vi "Organizing Tool.vi"() -> ()   [LabVIEW 2024]
uses:
  <userlib>/_OpenG.lib/file/file.llb/openg_file.lvlib
panel:
  in  "dest folders":i32(listbox)
  in  "root path":path
  in  "source folders":i32(listbox)
  in  "Delete Source Only":bool
  in  "Copy from Source":bool
  in  "Delete Source Dir?":bool=TRUE
  in  "Move and Delete Source":bool
  in  "dest files":i32(listbox)
  in  "source files":i32(listbox)
  in  "Quit":bool
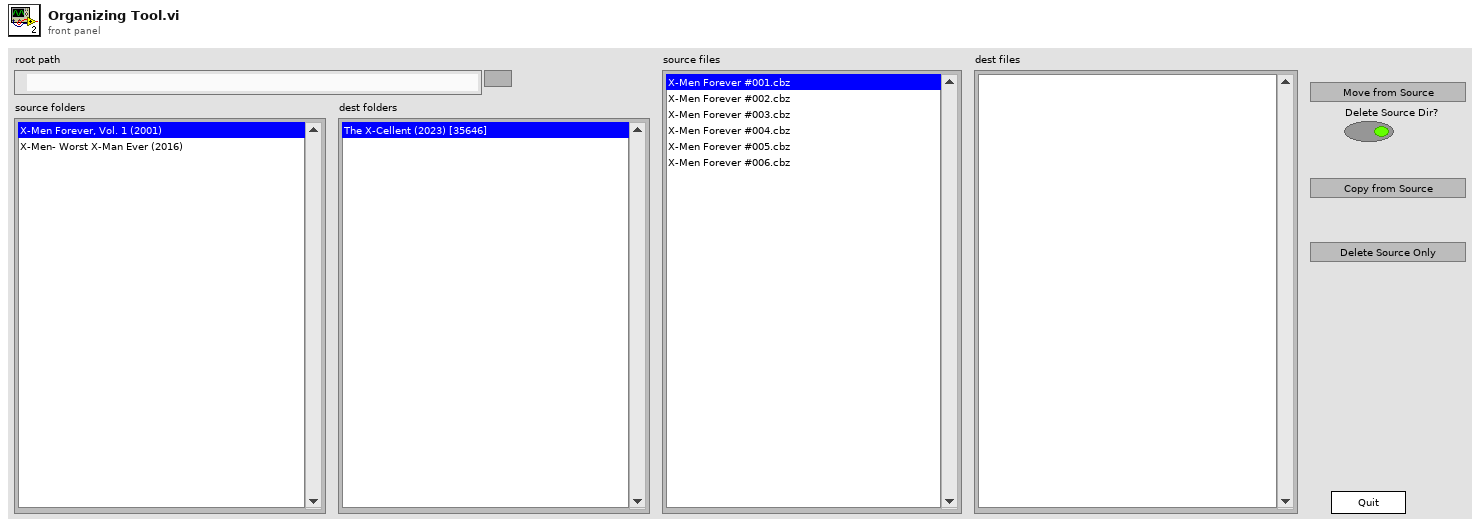
[diagram p1: front panel]
types:
  T1 = enum32{"Invalid", "Standard", "Closed", "Hidden", "Minimized", "Maximized"}
  T2 = enum32{"invalid app kind", "Development System", "Run Time System", "Student Edition", "Embedded LabVIEW", "Evaluation", "Custom"}
  T3 = cluster{"Core":cluster{"Current VI Reference":refnum<vi>, "Close Panel on Exit?":bool}, "source path":path, "dest path":path, "last source value":i32, "last dest value":i32}
  T4 = cluster{"Current VI Reference":refnum<vi>, "Close Panel on Exit?":bool}
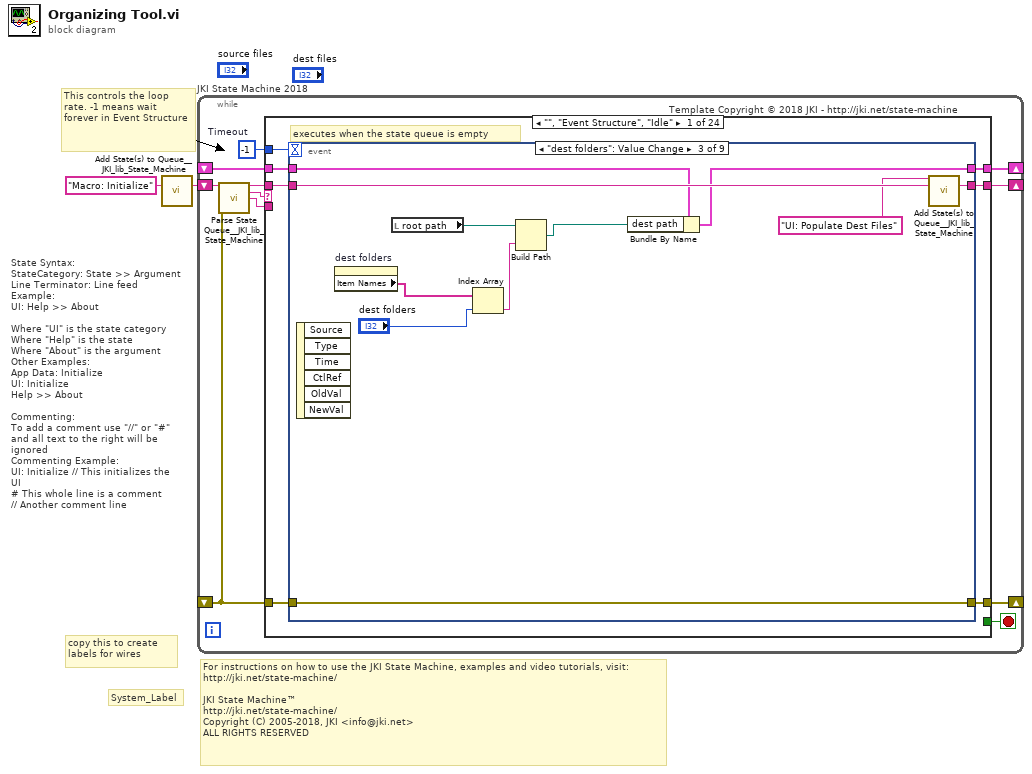
[diagram p0: block diagram]
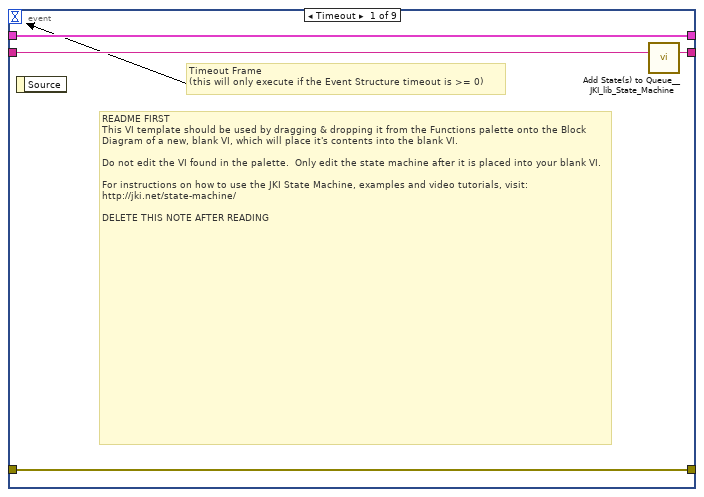
[diagram p2: hidden frame]
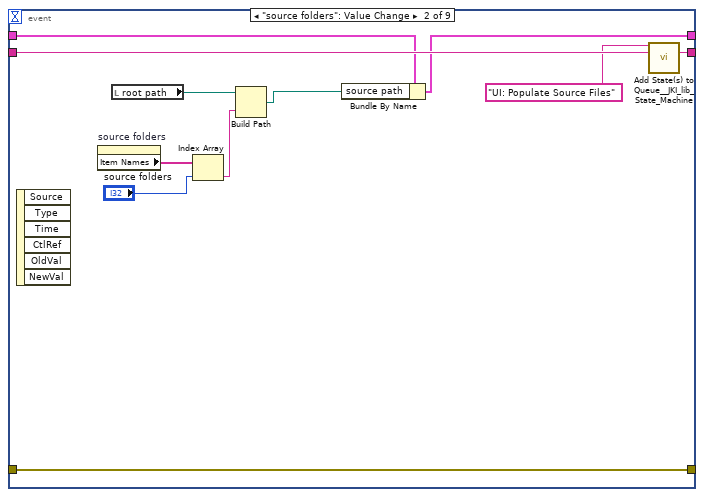
[diagram p3: hidden frame]
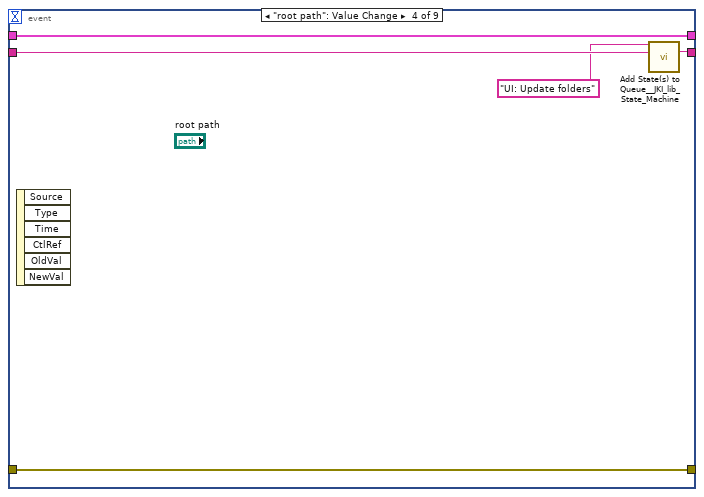
[diagram p4: hidden frame]
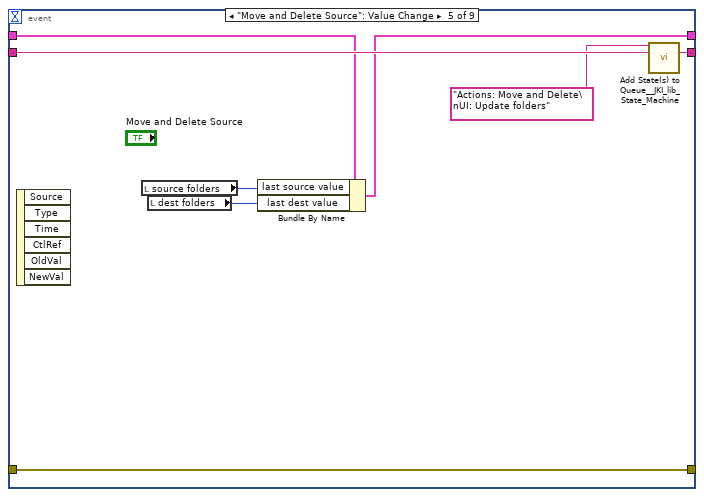
[diagram p5: hidden frame]
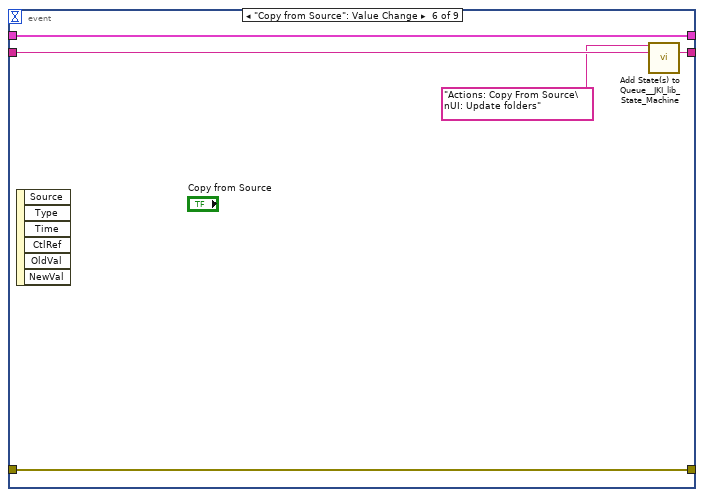
[diagram p6: hidden frame]
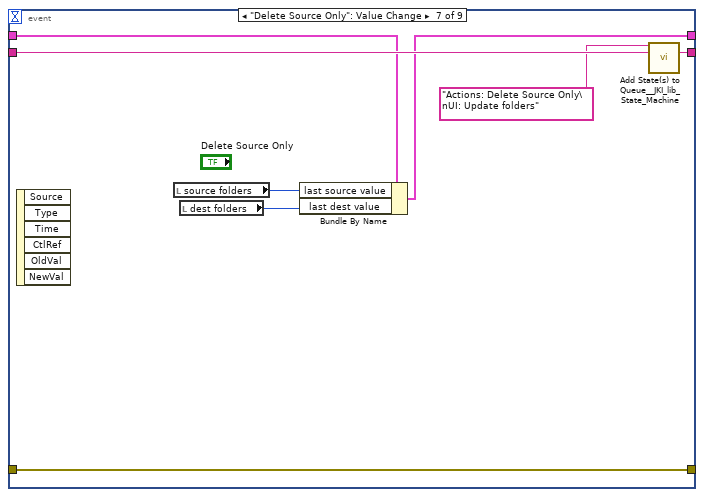
[diagram p7: hidden frame]
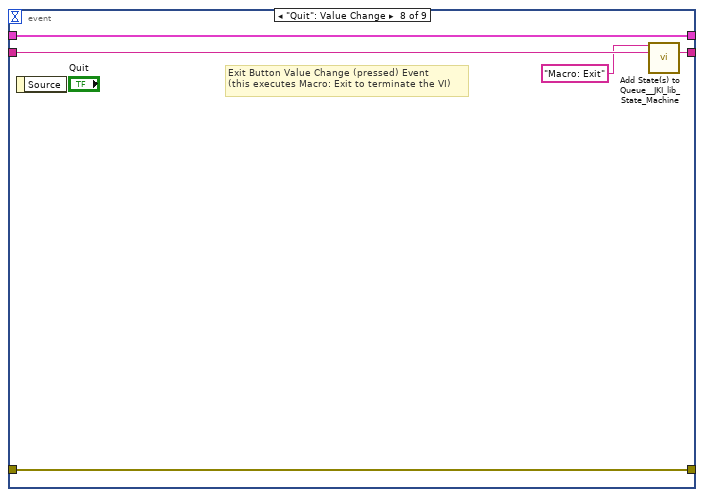
[diagram p8: hidden frame]
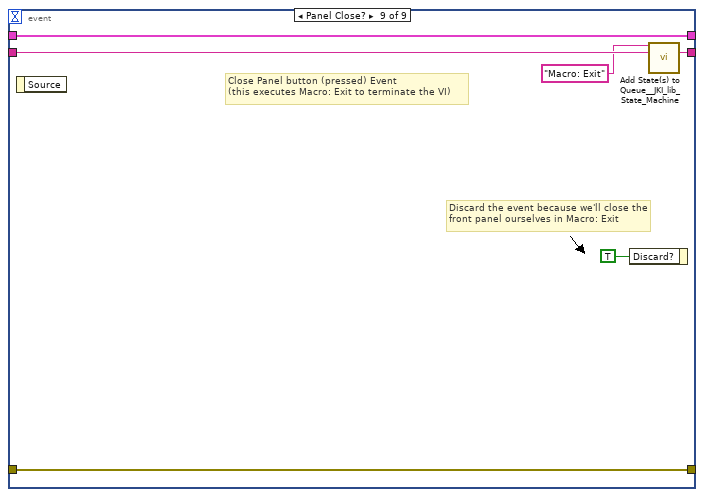
[diagram p9: hidden frame]
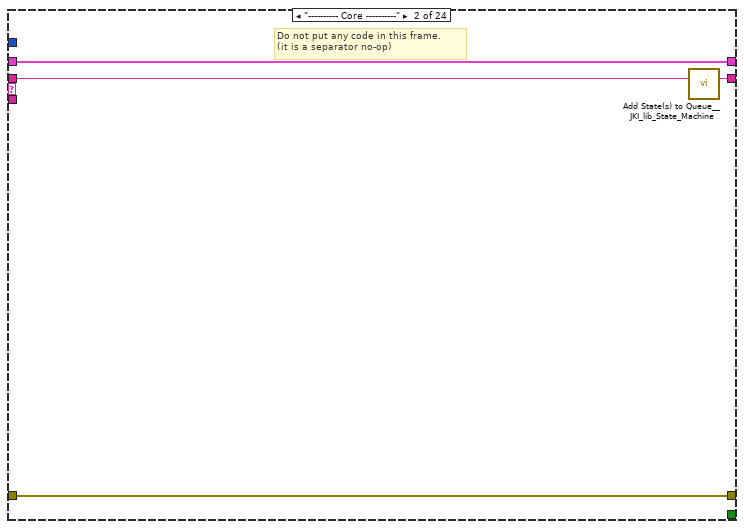
[diagram p10: hidden frame]
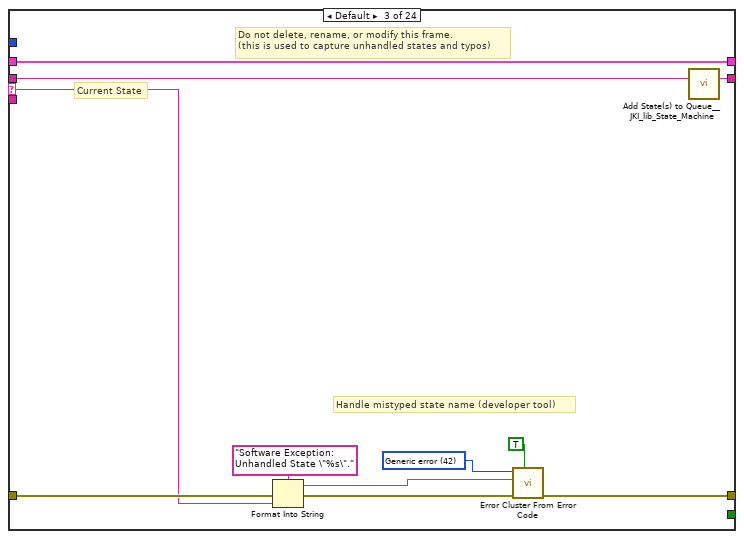
[diagram p11: hidden frame]
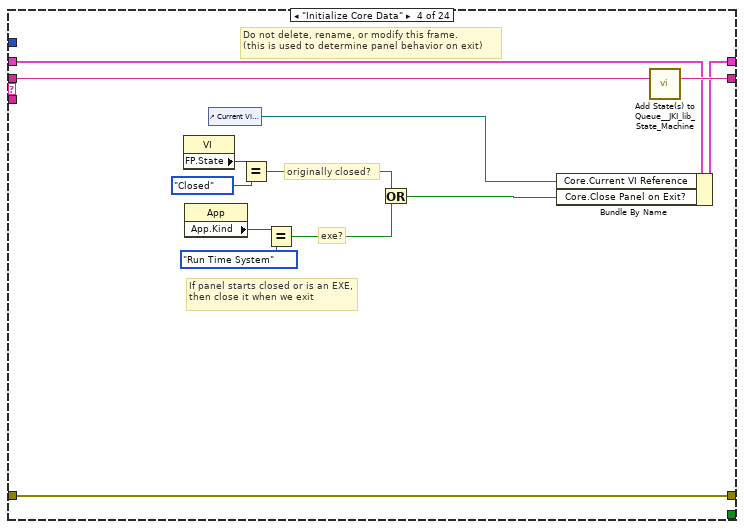
[diagram p12: hidden frame]
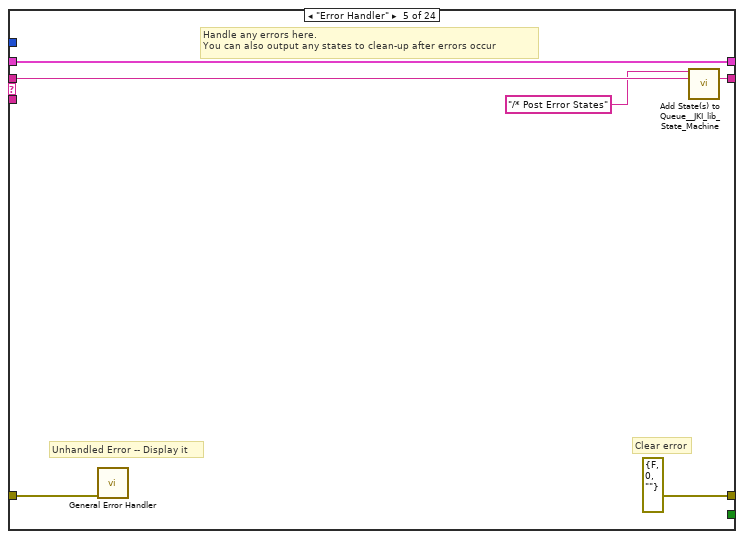
[diagram p13: hidden frame]
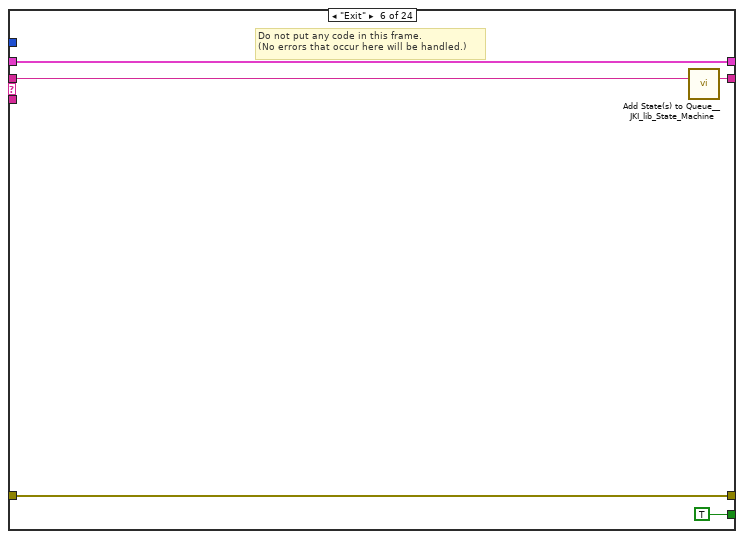
[diagram p14: hidden frame]
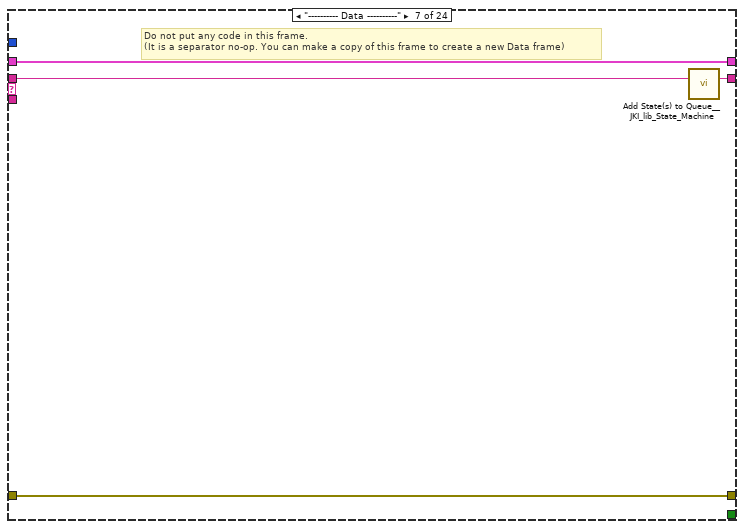
[diagram p15: hidden frame]
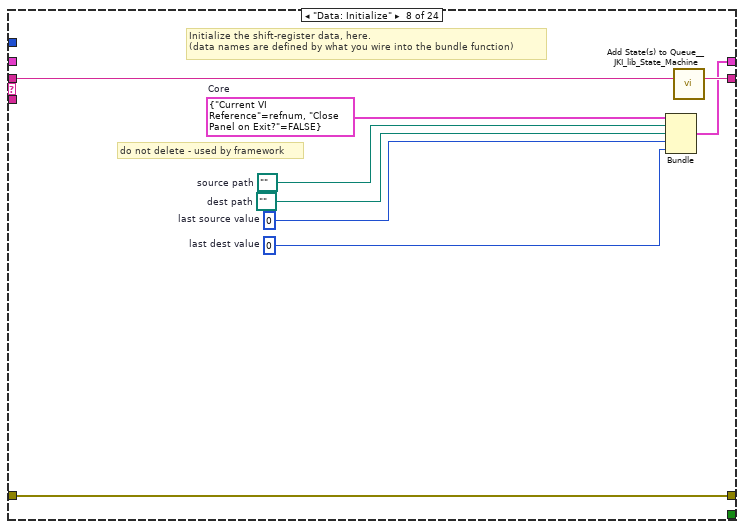
[diagram p16: hidden frame]
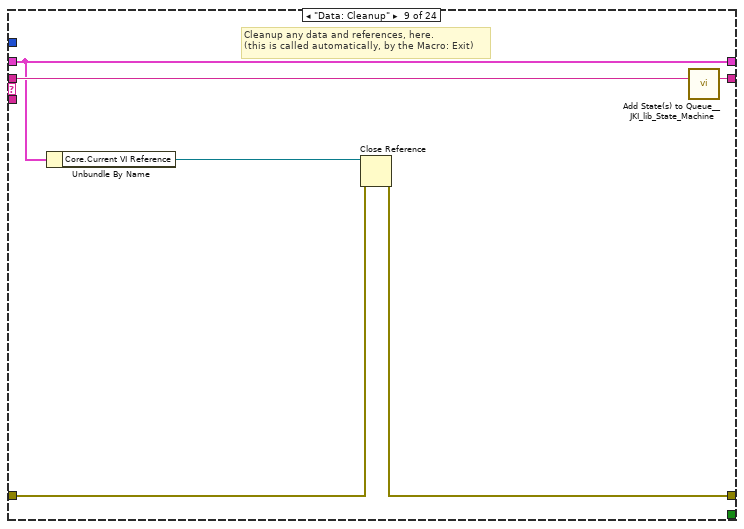
[diagram p17: hidden frame]
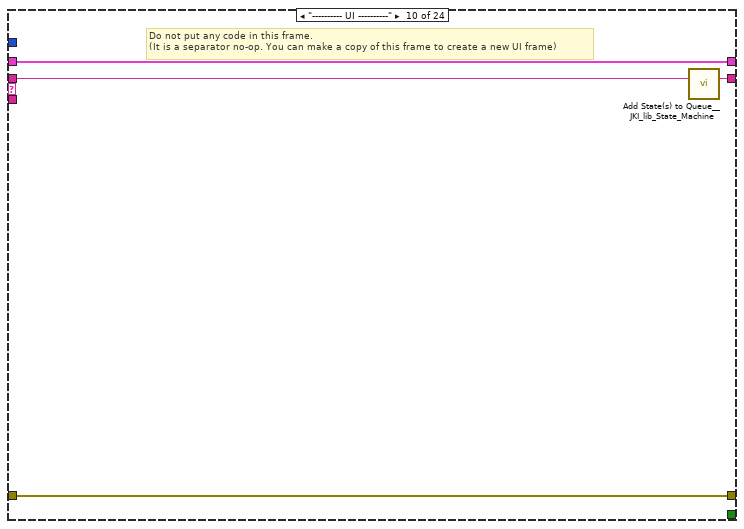
[diagram p18: hidden frame]
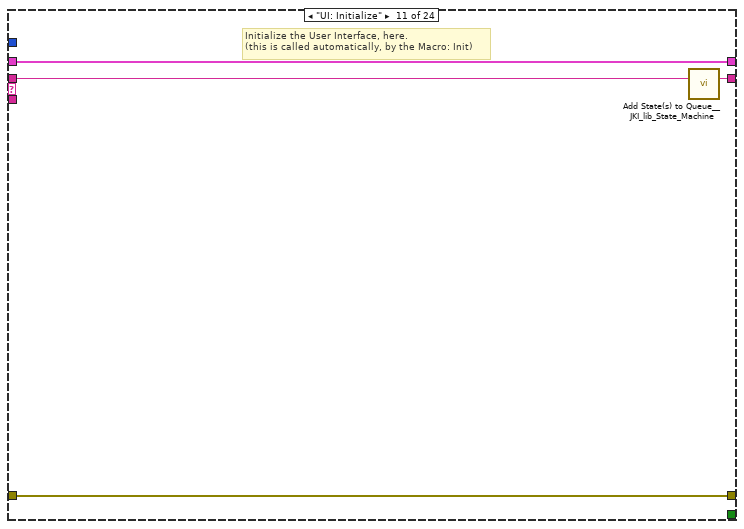
[diagram p19: hidden frame]
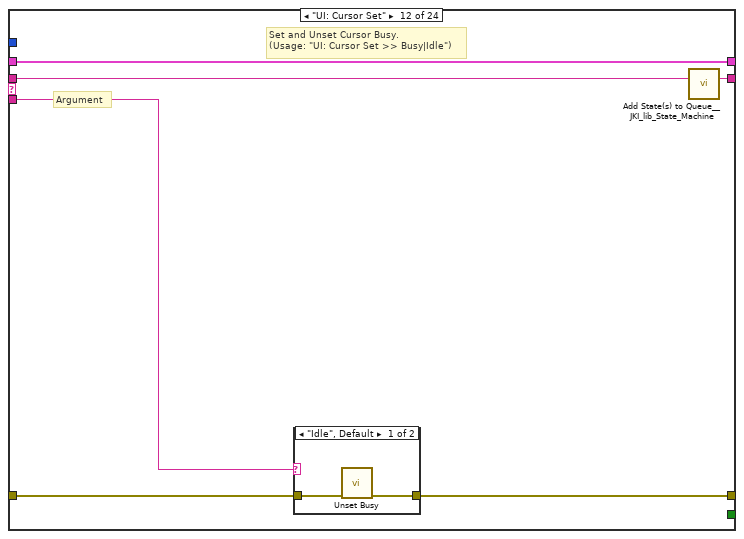
[diagram p20: hidden frame]
diagram:
  # "For instructions on how to use the JKI State Machine, examples and video tutorials, visit:\nhttp://jki.net/state-machine/\n\nJKI State Machine™\nhttp://jki.net/state-machine/\nCopyright (C) 2005-2018, JKI <info@jki.net>\nALL RIGHTS RESERVED"
  # "State Syntax:\nStateCategory: State >> Argument\nLine Terminator: Line feed\nExample:\nUI: Help >> About\n\nWhere \"UI\" is the state category\nWhere \"Help\" is the state\nWhere \"About\" is the argument\nOther Examples:\nApp Data: Initialize\nUI: Initialize\nHelp >> About\n\nCommenting:\nTo add a comment use \"//\" or \"#\" and all text to the right will be ignored\nCommenting Example:\nUI: Initialize // This initializes the UI\n# This whole line is a comment\n// Another comment line"
  # "copy this to create labels for wires"
  # "This controls the loop rate. -1 means wait forever in Event Structure"
  # "System_Label"
  n1 = call <vilib>:"Add State(s) to Queue__JKI_lib_State_Machine.vi"("State(s) in (\"\")"="Macro: Initialize") -> ("States Out"=w2:string)  [unwired: 14 in]
  n2 = while "JKI State Machine 2018" {
    shift-right: [w6] -> _
    shift-left: _ -> [w5]
    shift-right: [w9] -> _
    shift-left: _ -> [w3]
    shift-right: [w8] -> _
    shift-left: w2 -> [w10]
    stop <- w7 stop-if-true
    w4 = -1  # Timeout
    # "Template Copyright © 2018 JKI - http://jki.net/state-machine"
    n3 = call <vilib>:"Parse State Queue__JKI_lib_State_Machine.vi"("State Queue"=w10, "Error In (no error)"=w3) -> ("Remaining States"=w12:string, "Current State"=w13:string, "Arguments"=w11:string)  [unwired: 11 in]
    n4 = case shown="\"\", \"Event Structure\", \"Idle\"" w13 {
      selector: w13 -> [_ _ w88 _ _ _ _ _ _ _ _ _ _ _ _ _ _ _ _ _ _ _ _ _]
      tunnel: w12 -> [w20 w87 w92 w111 w117 w122 w126 w135 w141 w145 w149 w155 w166 w243 w260 w280 w284 w289 w299 w303 w311 w319 w326 w330]
      tunnel: w11 -> [_ _ _ _ _ _ _ _ _ _ _ w150 w160 _ _ _ _ _ _ _ _ _ _ _]
      tunnel: w5 -> [w18 w84 w90 w104 w114 w120 w123 _ w136 w142 w147 w153 w162 w242 w254 w279 w281 w286 w296 w300 w309 w317 w324 w327]
      tunnel: [w17 w85 w94 w108 errorcluster {"status"=FALSE, "code"=0, "source"=""} ("error out") w119 w124 w132 w137 w143 w146 w151 w163 w233 w246 w275 w282 w287 w297 w301 w306 w314 w321 w328] -> w9
      tunnel: w3 -> [w16 w85 w93 w108 w113 w119 w124 w132 w138 w143 w146 w152 w164 w240 w259 w277 w282 w287 w297 w301 w305 w313 w322 w328]
      tunnel: [w19 w86 w91 w110 w116 w121 w125 w134 w140 w144 w148 w154 w165 w243 w260 w280 w283 w288 w298 w302 w310 w318 w325 w329] -> w8
      tunnel: [_ _ _ _ _ TRUE _ _ _ _ _ _ _ _ _ _ _ _ _ _ _ _ _ _] -> w7
      tunnel: [w15 w84 w90 w109 w114 w120 w123 w133 w136 w142 w147 w153 w162 w242 w254 w279 w281 w286 w296 w300 w309 w317 w324 w327] -> w6
      tunnel: w4 -> [w14 _ _ _ _ _ _ _ _ _ _ _ _ _ _ _ _ _ _ _ _ _ _ _]
      frame "", "Event Structure", "Idle" {
        # "executes when the state queue is empty"
        n5 = event shown="[2] \"dest folders\": Value Change" {
          selector: _ -> [_ _ _ _ _ _ _ _ _]
          dyn-events: _ -> [_ _ _ _ _ _ _ _ _]
          timeout: w14 -> [_ _ _ _ _ _ _ _ _]
          tunnel: w20 -> [w24 w35 w46 w50 w58 w62 w71 w77 w83]
          tunnel: [w23 w34 w45 w49 w56 w60 w69 w76 w82] -> w19
          tunnel: w18 -> [w21 w33 w44 w51 w55 w63 w68 w74 w80]
          tunnel: [w22 w30 w41 w47 w59 w64 w72 w75 w81] -> w17
          tunnel: w16 -> [w22 w30 w41 w47 w59 w64 w72 w75 w81]
          tunnel: [w21 w32 w43 w51 w54 w63 w66 w74 w80] -> w15
          event Timeout {
            # "README FIRST\nThis VI template should be used by dragging & dropping it from the Functions palette onto the Block Diagram of a new, blank VI, which will place it's contents into the blank VI.\n\nDo not edit the VI found in the palette.  Only edit the state machine after it is placed into your blank VI.\n\nFor instructions on how to use the JKI State Machine, examples and video tutorials, visit:\nhttp://jki.net/state-machine/\n\nDELETE THIS NOTE AFTER READING"
            # "Timeout Frame\n(this will only execute if the Event Structure timeout is >= 0)"
            n6 = event-data() -> ()  [unwired: 1 in, 1 out]
            n7 = call <vilib>:"Add State(s) to Queue__JKI_lib_State_Machine.vi"("State(s) in (\"\")"=w24) -> ("States Out"=w23:string)  [unwired: 14 in]
          }
          event "source folders": Value Change {
            n8 = event-data() -> ()  [unwired: 1 in, 6 out]
            n9 = property on="source folders" class="LstBox (strict)"() -> ("Item Names"=w29:string[])  [unwired: 2 in, 2 out]
            n10 = local read "root path"() -> (w27:path)
            n11 = Index Array(array=w29, index="source folders") -> (element=w26:string)
            n12 = Build Path(base path=w27, name or relative path=w26) -> (appended path=w25:path)
            n13 = Bundle By Name(cluster=w33, "source path"=w25) -> (w32:T3)
            n14 = call <vilib>:"Add State(s) to Queue__JKI_lib_State_Machine.vi"("State(s) in Front (\"\")"="UI: Populate Source Files" ("State(s) in Front (\"\")"), "State(s) in (\"\")"=w35) -> ("States Out"=w34:string)  [unwired: 13 in]
          }
          event "dest folders": Value Change {
            n15 = event-data() -> ()  [unwired: 1 in, 6 out]
            n16 = property on="dest folders" class="LstBox (strict)"() -> ("Item Names"=w36:string[])  [unwired: 2 in, 2 out]
            n17 = local read "root path"() -> (w40:path)
            n18 = Index Array(array=w36, index="dest folders") -> (element=w39:string)
            n19 = Build Path(base path=w40, name or relative path=w39) -> (appended path=w38:path)
            n20 = Bundle By Name(cluster=w44, "dest path"=w38) -> (w43:T3)
            n21 = call <vilib>:"Add State(s) to Queue__JKI_lib_State_Machine.vi"("State(s) in Front (\"\")"="UI: Populate Dest Files" ("State(s) in Front (\"\")"), "State(s) in (\"\")"=w46) -> ("States Out"=w45:string)  [unwired: 13 in]
          }
          event "root path": Value Change {
            n22 = event-data() -> ()  [unwired: 1 in, 6 out]
            n23 = call <vilib>:"Add State(s) to Queue__JKI_lib_State_Machine.vi"("State(s) in Front (\"\")"="UI: Update folders" ("State(s) in Front (\"\")"), "State(s) in (\"\")"=w50) -> ("States Out"=w49:string)  [unwired: 13 in]
          }
          event "Move and Delete Source": Value Change {
            n24 = event-data() -> ()  [unwired: 1 in, 6 out]
            n25 = local read "source folders"() -> (w53:i32)
            n26 = local read "dest folders"() -> (w52:i32)
            n27 = Bundle By Name(cluster=w55, "last source value"=w53, "last dest value"=w52) -> (w54:T3)
            n28 = call <vilib>:"Add State(s) to Queue__JKI_lib_State_Machine.vi"("State(s) in Front (\"\")"="Actions: Move and Delete\nUI: Update folders" ("State(s) in Front (\"\")"), "State(s) in (\"\")"=w58) -> ("States Out"=w56:string)  [unwired: 13 in]
          }
          event "Copy from Source": Value Change {
            n29 = event-data() -> ()  [unwired: 1 in, 6 out]
            n30 = call <vilib>:"Add State(s) to Queue__JKI_lib_State_Machine.vi"("State(s) in Front (\"\")"="Actions: Copy From Source\nUI: Update folders" ("State(s) in Front (\"\")"), "State(s) in (\"\")"=w62) -> ("States Out"=w60:string)  [unwired: 13 in]
          }
          event "Delete Source Only": Value Change {
            n31 = event-data() -> ()  [unwired: 1 in, 6 out]
            n32 = local read "source folders"() -> (w67:i32)
            n33 = local read "dest folders"() -> (w65:i32)
            n34 = Bundle By Name(cluster=w68, "last source value"=w67, "last dest value"=w65) -> (w66:T3)
            n35 = call <vilib>:"Add State(s) to Queue__JKI_lib_State_Machine.vi"("State(s) in Front (\"\")"="Actions: Delete Source Only\nUI: Update folders" ("State(s) in Front (\"\")"), "State(s) in (\"\")"=w71) -> ("States Out"=w69:string)  [unwired: 13 in]
          }
          event "Quit": Value Change {
            # "Exit Button Value Change (pressed) Event\n(this executes Macro: Exit to terminate the VI)"
            n36 = event-data() -> ()  [unwired: 1 in, 1 out]
            n37 = call <vilib>:"Add State(s) to Queue__JKI_lib_State_Machine.vi"("State(s) in Front (\"\")"="Macro: Exit", "State(s) in (\"\")"=w77) -> ("States Out"=w76:string)  [unwired: 13 in]
          }
          event Panel Close? {
            # "Discard the event because we'll close the front panel ourselves in Macro: Exit"
            # "Close Panel button (pressed) Event\n(this executes Macro: Exit to terminate the VI)"
            n38 = event-data() -> ()  [unwired: 1 in, 1 out]
            n39 = event-data("Discard?"=TRUE) -> ()  [unwired: 1 in, 1 out]
            n40 = call <vilib>:"Add State(s) to Queue__JKI_lib_State_Machine.vi"("State(s) in Front (\"\")"="Macro: Exit", "State(s) in (\"\")"=w83) -> ("States Out"=w82:string)  [unwired: 13 in]
          }
        }
      }
      frame "---------- Core ----------" {
        # "Do not put any code in this frame.\n(it is a separator no-op)"
        n41 = call <vilib>:"Add State(s) to Queue__JKI_lib_State_Machine.vi"("State(s) in (\"\")"=w87) -> ("States Out"=w86:string)  [unwired: 14 in]
      }
      frame Default {
        w97 = 42 items=["No error", "Argument error", "Memory is full", "Out of zone", "End of file", "File already open", "Generic file I/O error", "File not found", "File permission error", "Disk is full", "Duplicate path", "Too many files open", "System feature not enabled", "Resource file not found", "Cannot add resource", "Resource not found", "Image not found", "Image memory error", "Pen does not exist", "Config type invalid", "Config token not found", "Config parse error", "Config memory error", "Bad external code format", "Bad external code offset", "External code not present", "Null window", "Destroy window error", "Null menu", "Print aborted", "Bad print record", "Print driver error", "Windows error during printing", "Memory error during printing", "Print dialog error", "Generic print error", "Invalid device refnum", "Device not found", "Device parameter error", "Device unit error", "Cannot open device", "Device call aborted", "Generic error", "Cancelled by user", "Object ID too low", "Object ID too high", "Object not in heap", "Unknown heap", "Unknown object (invalid DefProc)", "Unknown object (DefProc not in table)", "Message out of range", "Invalid (null) method", "Unknown message", "Manager call not supported", "Bad address", "Network operation in progress", "Network operation timed out", "Connection is busy", "Network attribute not supported", "Network error", "Address in use", "System out of memory", "Connection aborted", "Connection refused", "Not connected", "Already connected", "Connection closed", "Initialization error (interapplication manager)", "Bad occurrence", "Wait on unbound occurrence handler", "Occurrence queue overflow", "Datalog type conflict", "Unused", "Unrecognized type (interapplication manager)", "Memory corrupt", "Failed to make temporary DLL", "Old CIN version", "Drag socket not found", "Failed to load drop-object", "Failed to register OLE object", "Failed to release OLE object", "Format specifier type mismatch", "Unknown format specifier", "Too few format specifiers", "Too many format specifiers", "Scan failed", "Newer CIN version", "Error converting to variant", "Runtime menu error", "Password tampered", "Variant attribute not found", "Incompatible variant data type", "Event data is not available", "Event Store is not present", "Occurrence is not found", "Event Queue is not created", "Event info is not available", "Refnum passed is NULL", "Error retrieving Class GUID", "Error retrieving CoClass GUID", "Error retrieving TypeLib GUID.", "Bad built application magic bytes.", "Specific driver is different from the specific driver associated with the Logical Name.", "There is no session opened to the class driver.", "Max Error", "MAX - Error with config objects", "MAX - Error loading configuration", "MAX - Group not supported"]
        # "Current State"
        # "Do not delete, rename, or modify this frame.\n(this is used to capture unhandled states and typos)"
        # "Handle mistyped state name (developer tool)"
        n42 = Format Into String(format string="Software Exception: Unhandled State \"%s\"." ("message"), error in=w93, w88) -> (resulting string=w96:string, error out=w95:errorcluster)  [unwired: 1 in]
        n43 = call <vilib>:"Error Cluster From Error Code.vi"("show call chain? (False)"=TRUE, "error in (no error)"=w95, "error message (\"\")"=w96, "error code (0)"=w97) -> ("error out"=w94:errorcluster)  [unwired: 5 in]
        n44 = call <vilib>:"Add State(s) to Queue__JKI_lib_State_Machine.vi"("State(s) in (\"\")"=w92) -> ("States Out"=w91:string)  [unwired: 14 in]
      }
      frame "Initialize Core Data" {
        # "Do not delete, rename, or modify this frame.\n(this is used to determine panel behavior on exit)"
        # "originally closed?"
        # "exe?"
        # "If panel starts closed or is an EXE, then close it when we exit"
        n45 = property class="VI"() -> ("FP.State"=w101:T1)  [unwired: 2 in, 2 out]
        n46 = property class="App"() -> ("App.Kind"=w107:T2)  [unwired: 2 in, 2 out]
        n47 = control-ref of="Current VI Reference"() -> (w102:refnum<vi>)
        n48 = Equal?(x=w101, y=T1."Closed" ("Front Panel Window:State")) -> (x = y?=w99:bool)
        n49 = Equal?(x=w107, y=T2."Run Time System" ("Application:Kind")) -> (x = y?=w105:bool)
        n50 = Or(x=w99, y=w105) -> (x .or. y?=w103:bool)
        n51 = Bundle By Name(cluster=w104, "Core.Current VI Reference"=w102, "Core.Close Panel on Exit?"=w103) -> (w109:T3)
        n52 = call <vilib>:"Add State(s) to Queue__JKI_lib_State_Machine.vi"("State(s) in (\"\")"=w111) -> ("States Out"=w110:string)  [unwired: 14 in]
      }
      frame "Error Handler" {
        # "Unhandled Error -- Display it"
        # "Handle any errors here.\nYou can also output any states to clean-up after errors occur"
        # "Clear error"
        n53 = call <vilib>:"General Error Handler.vi"("error in (no error)"=w113) -> ()  [unwired: 10 in, 5 out]
        n54 = call <vilib>:"Add State(s) to Queue__JKI_lib_State_Machine.vi"("State(s) in Front (\"\")"="/* Post Error States", "State(s) in (\"\")"=w117) -> ("States Out"=w116:string)  [unwired: 13 in]
      }
      frame "Exit" {
        # "Do not put any code in this frame.\n(No errors that occur here will be handled.)"
        n55 = call <vilib>:"Add State(s) to Queue__JKI_lib_State_Machine.vi"("State(s) in (\"\")"=w122) -> ("States Out"=w121:string)  [unwired: 14 in]
      }
      frame "---------- Data ----------" {
        # "Do not put any code in this frame.\n(It is a separator no-op. You can make a copy of this frame to create a new Data frame)"
        n56 = call <vilib>:"Add State(s) to Queue__JKI_lib_State_Machine.vi"("State(s) in (\"\")"=w126) -> ("States Out"=w125:string)  [unwired: 14 in]
      }
      frame "Data: Initialize" {
        w127 = 0  # last dest value
        w128 = 0  # last source value
        w129 = T4 {"Current VI Reference"=refnum, "Close Panel on Exit?"=FALSE}  # Core
        w131 = path ""  # source path
        w130 = path ""  # dest path
        # "do not delete - used by framework"
        # "Initialize the shift-register data, here.\n(data names are defined by what you wire into the bundle function)"
        n57 = Bundle("Core"=w129, "source path"=w131, "dest path"=w130, "last source value"=w128, "last dest value"=w127) -> (w133:T3)  [unwired: 1 in]
        n58 = call <vilib>:"Add State(s) to Queue__JKI_lib_State_Machine.vi"("State(s) in (\"\")"=w135) -> ("States Out"=w134:string)  [unwired: 14 in]
      }
      frame "Data: Cleanup" {
        # "Cleanup any data and references, here.\n(this is called automatically, by the Macro: Exit)"
        n59 = Unbundle By Name(w136) -> ("Core.Current VI Reference"=w139:refnum<vi>)
        n60 = Close Reference(reference=w139, error in (no error)=w138) -> (error out=w137:errorcluster)
        n61 = call <vilib>:"Add State(s) to Queue__JKI_lib_State_Machine.vi"("State(s) in (\"\")"=w141) -> ("States Out"=w140:string)  [unwired: 14 in]
      }
      frame "---------- UI ----------" {
        # "Do not put any code in this frame.\n(It is a separator no-op. You can make a copy of this frame to create a new UI frame)"
        n62 = call <vilib>:"Add State(s) to Queue__JKI_lib_State_Machine.vi"("State(s) in (\"\")"=w145) -> ("States Out"=w144:string)  [unwired: 14 in]
      }
      frame "UI: Initialize" {
        # "Initialize the User Interface, here.\n(this is called automatically, by the Macro: Init)"
        n63 = call <vilib>:"Add State(s) to Queue__JKI_lib_State_Machine.vi"("State(s) in (\"\")"=w149) -> ("States Out"=w148:string)  [unwired: 14 in]
      }
      frame "UI: Cursor Set" {
        # "Argument"
        # "Set and Unset Cursor Busy.\n(Usage: \"UI: Cursor Set >> Busy|Idle\")"
        n64 = case shown="\"Idle\", Default" w150 {
          tunnel: w152 -> [w157 w159]
          tunnel: [w156 w158] -> w151
          frame "Idle", Default {
            n65 = call <vilib>:"Unset Busy.vi"("error in (no error)"=w157) -> ("error out"=w156:errorcluster)  [unwired: 10 in]
          }
          frame "Busy" {
            n66 = call <vilib>:"Set Busy.vi"("error in (no error)"=w159) -> ("error out"=w158:errorcluster)  [unwired: 9 in, 1 out]
          }
        }
        n67 = call <vilib>:"Add State(s) to Queue__JKI_lib_State_Machine.vi"("State(s) in (\"\")"=w155) -> ("States Out"=w154:string)  [unwired: 14 in]
      }
      frame "UI: Front Panel State" {
        # "Argument"
        # "Set Front Panel Open or Closed\n(Usage: \"UI: Front Panel State >> Open|Close\")"
        n68 = Unbundle By Name(w162) -> ("Core.Current VI Reference"=w161:refnum<vi>)
        n69 = case shown="\"Minimize\", \"Minimized\"" w160 {
          tunnel: w164 -> [w172 w187 w198 w211 w224]
          tunnel: [w174 w188 w200 w213 w226] -> w163
          tunnel: w161 -> [w173 w185 w199 w212 w225]
          frame "Open", "Standard", Default {
            w167 = T1."Standard" ("State")
            n70 = property class="VI"(reference=w173, error in=w172) -> (reference out=w170:refnum<vi>, error out=w171:errorcluster, "FP.State"=w169:T1)
            n71 = Not Equal?(x=w169, y=w167) -> (x != y?=w168:bool)
            n72 = case shown="True" w168 {
              tunnel: [w178 w180] -> w174
              tunnel: w171 -> [w177 w180]
              tunnel: w170 -> [w176 _]
              tunnel: w167 -> [w175 _]
              frame True {
                n73 = invoke class="VI" method="FP.Open"(reference=w176, error in=w177, "Activate"=TRUE, "State"=w175) -> (error out=w178:errorcluster)  [unwired: 1 in, 4 out]
              }
              frame False {
              }
            }
          }
          frame "Close", "Closed" {
            n74 = property class="VI"(reference=w185, error in=w187) -> (reference out=w184:refnum<vi>, error out=w186:errorcluster, "FP.State"=w182:T1)
            n75 = Not Equal?(x=w182, y=T1."Closed" ("Front Panel Window:State")) -> (x != y?=w181:bool)
            n76 = case shown="True" w181 {
              tunnel: [w189 w192] -> w188
              tunnel: w186 -> [w189 w191]
              tunnel: w184 -> [_ w190]
              frame False {
              }
              frame True {
                n77 = invoke class="VI" method="FP.Close"(reference=w190, error in=w191) -> (error out=w192:errorcluster)  [unwired: 1 in, 2 out]
              }
            }
          }
          frame "Hidden", "Hide" {
            w193 = T1."Hidden" ("State")
            n78 = property class="VI"(reference=w199, error in=w198) -> (reference out=w196:refnum<vi>, error out=w197:errorcluster, "FP.State"=w195:T1)
            n79 = Not Equal?(x=w195, y=w193) -> (x != y?=w194:bool)
            n80 = case shown="True" w194 {
              tunnel: [w204 w205] -> w200
              tunnel: w197 -> [w203 w205]
              tunnel: w196 -> [w202 _]
              tunnel: w193 -> [w201 _]
              frame True {
                n81 = invoke class="VI" method="FP.Open"(reference=w202, error in=w203, "State"=w201) -> (error out=w204:errorcluster)  [unwired: 2 in, 4 out]
              }
              frame False {
              }
            }
          }
          frame "Minimize", "Minimized" {
            w206 = T1."Minimized" ("State")
            n82 = property class="VI"(reference=w212, error in=w211) -> (reference out=w209:refnum<vi>, error out=w210:errorcluster, "FP.State"=w208:T1)
            n83 = Not Equal?(x=w208, y=w206) -> (x != y?=w207:bool)
            n84 = case shown="True" w207 {
              tunnel: [w217 w218] -> w213
              tunnel: w210 -> [w216 w218]
              tunnel: w209 -> [w215 _]
              tunnel: w206 -> [w214 _]
              frame True {
                n85 = invoke class="VI" method="FP.Open"(reference=w215, error in=w216, "State"=w214) -> (error out=w217:errorcluster)  [unwired: 2 in, 4 out]
              }
              frame False {
              }
            }
          }
          frame "Maximize", "Maximized" {
            w219 = T1."Maximized" ("State")
            n86 = property class="VI"(reference=w225, error in=w224) -> (reference out=w222:refnum<vi>, error out=w223:errorcluster, "FP.State"=w221:T1)
            n87 = Not Equal?(x=w221, y=w219) -> (x != y?=w220:bool)
            n88 = case shown="True" w220 {
              tunnel: [w230 w231] -> w226
              tunnel: w223 -> [w229 w231]
              tunnel: w222 -> [w228 _]
              tunnel: w219 -> [w227 _]
              frame True {
                n89 = invoke class="VI" method="FP.Open"(reference=w228, error in=w229, "State"=w227) -> (error out=w230:errorcluster)  [unwired: 2 in, 4 out]
              }
              frame False {
              }
            }
          }
        }
        n90 = call <vilib>:"Add State(s) to Queue__JKI_lib_State_Machine.vi"("State(s) in (\"\")"=w166) -> ("States Out"=w165:string)  [unwired: 14 in]
      }
      frame "UI: Populate Source Files" {
        n91 = Unbundle By Name(w242) -> ("source path"=w241:path)
        n92 = List Folder(path=w241, error in=w240) -> (filenames=w237:string[], folder names=w236:string[], error out=w239:errorcluster)  [unwired: 2 in, 1 out]
        n93 = Build Array (concatenate)(w236, w237) -> (w235:string[])
        n94 = property on="source files" class="LstBox (strict)"(error in=w239, "Item Names"=w235, "Value"=-1 ("source files")) -> (error out=w238:errorcluster)  [unwired: 1 in, 1 out]
        n95 = call <vilib>:"Clear Errors.vi"("error in (no error)"=w238, "specific error code to clear (0: all)"=1430) -> ("error out"=w233:errorcluster)  [unwired: 4 in, 1 out]
      }
      frame "UI: Update folders" {
        n96 = local read "root path"() -> (w252:path)
        n97 = List Folder(path=w252, error in=w259) -> (folder names=w257:string[], error out=w258:errorcluster)  [unwired: 2 in, 2 out]
        n98 = for {
          tunnel: w257 -> [w266] mode=indexing
          tunnel: [w266] -> w255 mode=indexing if=w268
          tunnel: [w266] -> w256 mode=indexing if=w263
          tunnel: w252 -> [w267]
          n99 = Match Pattern(string=w266, regular expression="\\[") -> (offset past match=w269:i32)  [unwired: 1 in, 3 out]
          n100 = Build Path(base path=w267, name or relative path=w266) -> (appended path=w265:path)
          n101 = Less Than 0?(x=w269) -> (x < 0?=w268:bool)
          n102 = Not(x=w268) -> (.not. x?=w261:bool)
          n103 = List Folder(path=w265) -> (filenames=w264:string[])  [unwired: 3 in, 3 out]
          n104 = Empty Array?(array=w264) -> (empty?=w262:bool)
          n105 = And(x=w261, y=w262) -> (x .and. y?=w263:bool)
        }
        n106 = Unbundle By Name(w254) -> ("last source value"=w253:i32, "last dest value"=w251:i32)
        n107 = property on="source folders" class="LstBox (strict)"(error in=w258, "Item Names"=w255) -> (error out=w250:errorcluster)  [unwired: 1 in, 1 out]
        n108 = property on="dest folders" class="LstBox (strict)"(error in=w258, "Item Names"=w256) -> (error out=w249:errorcluster)  [unwired: 1 in, 1 out]
        n109 = property on="dest folders" class="LstBox (strict)"(error in=w249, "Val(Sgnl)"=w251) -> (error out=w247:errorcluster)  [unwired: 1 in, 1 out]
        n110 = property on="source folders" class="LstBox (strict)"(error in=w250, "Val(Sgnl)"=w253) -> (error out=w248:errorcluster)  [unwired: 1 in, 1 out]
        n111 = Merge Errors(w248, w247) -> (w245:errorcluster)
        n112 = call <vilib>:"Clear Errors.vi"("error in (no error)"=w245, "specific error code to clear (0: all)"=1430) -> ("error out"=w246:errorcluster)  [unwired: 4 in, 1 out]
      }
      frame "UI: Populate Dest Files" {
        n113 = Unbundle By Name(w279) -> ("dest path"=w278:path)
        n114 = List Folder(path=w278, error in=w277) -> (filenames=w272:string[], folder names=w273:string[], error out=w276:errorcluster)  [unwired: 2 in, 1 out]
        n115 = Build Array (concatenate)(w273, w272) -> (w271:string[])
        n116 = property on="dest files" class="LstBox (strict)"(error in=w276, "Item Names"=w271, "Value"=-1 ("dest files")) -> (error out=w275:errorcluster)  [unwired: 1 in, 1 out]
      }
      frame "---------- Macro ----------" {
        # "Do not put any code in this frame.\n(It is a separator no-op. You can make a copy of this frame to create a new Macro frame)"
        n117 = call <vilib>:"Add State(s) to Queue__JKI_lib_State_Machine.vi"("State(s) in (\"\")"=w284) -> ("States Out"=w283:string)  [unwired: 14 in]
      }
      frame "Macro: Initialize" {
        w285 = "Data: Initialize\nInitialize Core Data\nUI: Initialize\nUI: Front Panel State >> Open"  # Data: Initialize Initialize Core Data UI: Initialize UI: Front Panel State >> Open
        # "Initialization Macro\n(This is called once, when the VI starts)"
        n118 = call <vilib>:"Add State(s) to Queue__JKI_lib_State_Machine.vi"("State(s) in Front (\"\")"=w285, "State(s) in (\"\")"=w289) -> ("States Out"=w288:string)  [unwired: 13 in]
      }
      frame "Macro: Exit" {
        # "Exit Macro\n(This is called once, when the VI exits)"
        n119 = Unbundle By Name(w296) -> ("Core.Close Panel on Exit?"=w295:bool)
        n120 = Select(t="UI: Front Panel State >> Close", s=w295, f="") -> (s? t:f=w292:string)
        n121 = call <vilib>:"Add State(s) to Queue__JKI_lib_State_Machine.vi"("State(s) in (\"\")"=w292, "State(s) at Back (\"\")"="Data: Cleanup\nExit") -> ("States Out"=w290:string)  [unwired: 13 in]
        n122 = call <vilib>:"Add State(s) to Queue__JKI_lib_State_Machine.vi"("State(s) in Front (\"\")"=w290, "State(s) in (\"\")"=w299) -> ("States Out"=w298:string)  [unwired: 13 in]
      }
      frame "---------- Actions ----------" {
        # "Template Separator\n(You can make a copy of, or modify, this frame)"
        n123 = call <vilib>:"Add State(s) to Queue__JKI_lib_State_Machine.vi"("State(s) in (\"\")"=w303) -> ("States Out"=w302:string)  [unwired: 14 in]
      }
      frame "Actions: Move and Delete" {
        n124 = Unbundle By Name(w309) -> ("source path"=w308:path, "dest path"=w307:path)
        n125 = call "MoveFilesRecursively.vi"("Delete Source Dir?"="Delete Source Dir?", "error in"=w305, "Dest Path"=w307, "Source Path"=w308) -> ("error out"=w306:errorcluster)  [unwired: 7 in]
        n126 = call <vilib>:"Add State(s) to Queue__JKI_lib_State_Machine.vi"("State(s) in (\"\")"=w311) -> ("States Out"=w310:string)  [unwired: 14 in]
      }
      frame "Actions: Copy From Source" {
        w312 = FALSE ("Delete Source Dir?")
        n127 = Unbundle By Name(w317) -> ("source path"=w316:path, "dest path"=w315:path)
        n128 = call "MoveFilesRecursively.vi"("Delete Source files?"=w312, "Delete Source Dir?"=w312, "error in"=w313, "Dest Path"=w315, "Source Path"=w316) -> ("error out"=w314:errorcluster)  [unwired: 6 in]
        n129 = call <vilib>:"Add State(s) to Queue__JKI_lib_State_Machine.vi"("State(s) in (\"\")"=w319) -> ("States Out"=w318:string)  [unwired: 14 in]
      }
      frame "Actions: Delete Source Only" {
        w320 = TRUE ("Recursive? (FALSE)")
        n130 = Unbundle By Name(w324) -> ("source path"=w323:path)
        n131 = call <userlib>:"Delete Recursive__ogtk.vi"("error in (no error)"=w322, "Ignore Read-Only? (FALSE)"=w320, "Recursive? (FALSE)"=w320, "Path"=w323) -> ("error out"=w321:errorcluster)  [unwired: 6 in, 1 out]
        n132 = call <vilib>:"Add State(s) to Queue__JKI_lib_State_Machine.vi"("State(s) in (\"\")"=w326) -> ("States Out"=w325:string)  [unwired: 14 in]
      }
      frame "New Category: 2" {
        # "Your code here.\n(You can make a copy of, or modify, this frame)"
        n133 = call <vilib>:"Add State(s) to Queue__JKI_lib_State_Machine.vi"("State(s) in (\"\")"=w330) -> ("States Out"=w329:string)  [unwired: 14 in]
      }
    }
  }
